vi "Phasor Explorer Set Graph Properties.vi"(6 "Max Legend Size (8)":i32[](array[numeric]), 8 "Error In":errorcluster, 9 "# Preserved PLots":i32[](array[numeric]), 10 "Metadata Type":variant[](array[variant]), 11 "XY Graph Ref Array":refnum<vi>[](array[refnum])) -> (0 "Error Out":errorcluster)   [LabVIEW 2019]
uses:
  Arrays/Linear Ramp End Options.ctl
  Graphs/XY Graph/XY Graph Add-Ons.lvlib
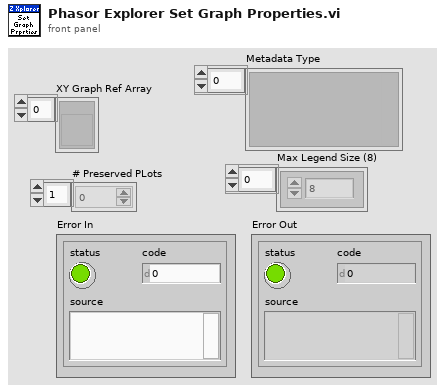
[diagram p1: front panel]
types:
  T1 = typedef "Linear Ramp End Options.ctl" = enum16{"Include Min/Exclude Max", "Exclude Min/Include Max", "Include Both Ends", "Exclude Both Ends"}
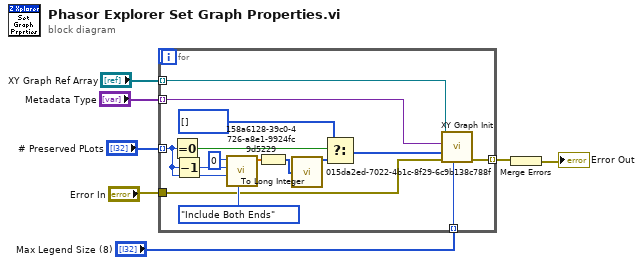
[diagram p0: block diagram]
diagram:
  n1 = for {
    tunnel: "XY Graph Ref Array" -> [w12] mode=indexing
    tunnel: "Error In" -> [w11]
    tunnel: "# Preserved PLots" -> [w21] mode=indexing
    tunnel: "Max Legend Size (8)" -> [w10] mode=indexing
    tunnel: [w9] -> w2 mode=indexing
    tunnel: "Metadata Type" -> [w8] mode=indexing
    n2 = Equal To 0?(x=w21) -> (x = 0?=w19:bool)
    n3 = Decrement(x=w21) -> (x-1=w20:i32)
    n4 = call "158a6128-39c0-4726-a8e1-9924fc9d5229.vi"("Options"=Linear_Ramp_End_Options."Include Both Ends", "# Steps (1)"=w21, "End (1)"=w20, "Start (0)"=0 ("Numeric")) -> ("Ramp"=w18:dbl[])  [unwired: 5 in, 2 out]
    n5 = To Long Integer(number=w18) -> (32bit integer=w16:i32[])
    n6 = call "015da2ed-7022-4b1c-8f29-6c9b138c788f.vi"("Input Array"=w16) -> ("Output Array"=w14:i32[])  [unwired: 1 out]
    n7 = Select(t=i32[] [] ("Numeric"), s=w19, f=w14) -> (s? t:f=w13:i32[])
    n8 = call "XY Graph Init.vi"("Max Legend Size (8)"=w10, "Error In"=w11, "Plots to Skip (none)"=w13, "Metadata Type"=w8, "XYGraph in"=w12) -> ("Error Out"=w9:errorcluster)  [unwired: 6 in]
  }
  n9 = Merge Errors(w2) -> (→"Error Out":errorcluster)
